vi "CH3_Save_Header_Python.vi"() -> ()   [LabVIEW 2018]
uses:
  RxTx/RxTx.lvclass
  Save Image/Save Image.lvclass
panel:
  out "error out":errorcluster
  in  "Save Image out":refnum<class "Save Image.lvclass">
  in  "RxTx.lvclass":refnum<class "RxTx.lvclass">
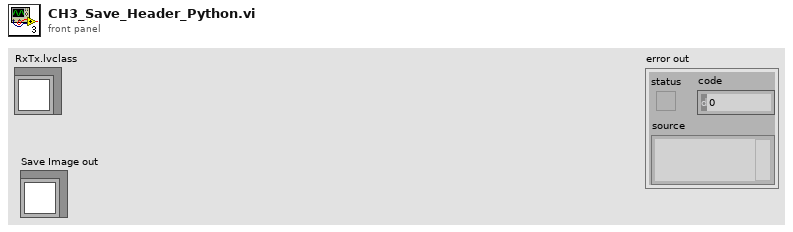
[diagram p1: front panel]
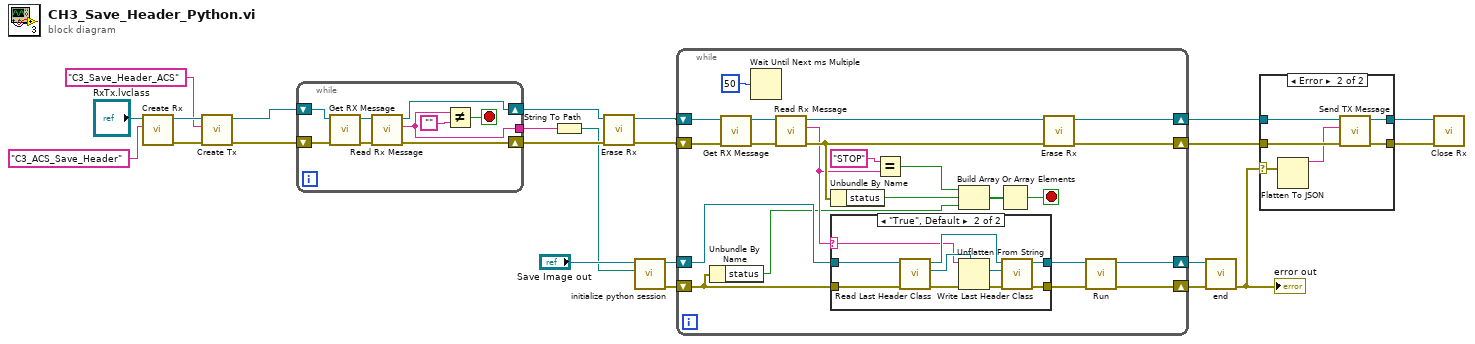
[diagram p0: block diagram]
diagram:
  n1 = call "Create Rx.vi"("Reader Name"="C3_ACS_Save_Header", "RxTx in"="RxTx.lvclass") -> ("error out"=w2:errorcluster, "RxTx out"=w5:refnum<class "RxTx.lvclass">)  [unwired: 8 in]
  n2 = call "Create Tx.vi"("error in (no error)"=w2, "Writer Name"="C3_Save_Header_ACS" ("Reader Name"), "RxTx in"=w5) -> ("error out"=w3:errorcluster, "RxTx out"=w4:refnum<class "RxTx.lvclass">)  [unwired: 7 in]
  n3 = while {
    shift-right: [w30] -> w16
    shift-left: w3 -> [w32]
    shift-right: [w29] -> w13
    shift-left: w4 -> [w27]
    tunnel: [w24] -> w11
    stop <- w25 stop-if-true
    n4 = call "Get RX Message.vi"("error in (no error)"=w32, "RxTx in"=w27) -> ("error out"=w31:errorcluster, "RxTx out"=w28:refnum<class "RxTx.lvclass">)  [unwired: 8 in]
    n5 = call "Read Rx Message.vi"("error in (no error)"=w31, "RxTx in"=w28) -> ("error out"=w30:errorcluster, "Rx Message"=w24:string, "RxTx out"=w29:refnum<class "RxTx.lvclass">)  [unwired: 7 in]
    n6 = Not Equal?(x=w24, y="") -> (x != y?=w25:bool)
  }
  n7 = String To Path(string=w11) -> (path=w12:path)
  n8 = call "Erase Rx.vi"("error in (no error)"=w16, "RxTx in"=w13) -> ("error out"=w15:errorcluster, "RxTx out"=w14:refnum<class "RxTx.lvclass">)  [unwired: 8 in]
  n9 = call "initialize python session.vi"("Optional Path to Python.exe"=w12, "Save Image in"="Save Image out") -> ("error out"=w20:errorcluster, "Save Image out"=w21:refnum<class "Save Image.lvclass">)  [unwired: 8 in]
  n10 = while {
    shift-right: [w42] -> w9
    shift-left: w15 -> [w53]
    shift-right: [w43] -> w10
    shift-left: w14 -> [w54]
    shift-right: [w45] -> w18
    shift-left: w21 -> [w47]
    shift-right: [w46] -> w17
    shift-left: w20 -> [w38]
    stop <- w33 stop-if-true
    n11 = Unbundle By Name(w38) -> ("status"=w37:bool)
    n12 = call "Get RX Message.vi"("error in (no error)"=w53, "RxTx in"=w54) -> ("error out"=w51:errorcluster, "RxTx out"=w52:refnum<class "RxTx.lvclass">)  [unwired: 8 in]
    n13 = Wait Until Next ms Multiple(millisecond multiple=u32 50) -> ()  [unwired: 1 out]
    n14 = call "Read Rx Message.vi"("error in (no error)"=w51, "RxTx in"=w52) -> ("error out"=w41:errorcluster, "Rx Message"=w39:string, "RxTx out"=w44:refnum<class "RxTx.lvclass">)  [unwired: 7 in]
    n15 = Unbundle By Name(w41) -> ("status"=w36:bool)
    n16 = case shown="\"True\", Default" w39 {
      selector: w39 -> [_ w57]
      tunnel: [w56 w58] -> w49
      tunnel: [w55 w59] -> w48
      tunnel: w38 -> [w55 w62]
      tunnel: w47 -> [w56 w63]
      frame "", "STOP" {
      }
      frame "True", Default {
        n17 = call "Read Last Header Class.vi"("error in (no error)"=w62, "Save Image in"=w63) -> ("error out"=w61:errorcluster, "Simulated_Header.lvclass"=w66:refnum<class "Simulated_Header.lvclass">, "Save Image out"=w64:refnum<class "Save Image.lvclass">)  [unwired: 7 in]
        n18 = Unflatten From String(type=w66, binary string=w57, error in (no error)=w61) -> (value=w65:refnum<class "Simulated_Header.lvclass">, error out=w60:errorcluster)  [unwired: 2 in, 1 out]
        n19 = call "Write Last Header Class.vi"("error in (no error)"=w60, "Simulated_Header.lvclass"=w65, "Save Image in"=w64) -> ("error out"=w59:errorcluster, "Save Image out"=w58:refnum<class "Save Image.lvclass">)  [unwired: 7 in]
      }
    }
    n20 = Equal?(x="STOP" ("Reader Name"), y=w39) -> (x = y?=w35:bool)
    n21 = Build Array(w35, w36, w37) -> (w34:bool[])
    n22 = Or Array Elements(Boolean array=w34) -> (logical OR=w33:bool)
    n23 = call "Erase Rx.vi"("error in (no error)"=w41, "RxTx in"=w44) -> ("error out"=w42:errorcluster, "RxTx out"=w43:refnum<class "RxTx.lvclass">)  [unwired: 8 in]
    n24 = call "Run.vi"("error in (no error)"=w48, "Save Image in"=w49) -> ("error out"=w46:errorcluster, "Save Image out"=w45:refnum<class "Save Image.lvclass">)  [unwired: 8 in]
  }
  n25 = call "end.vi"("error in (no error)"=w17, "Save Image in"=w18) -> ("error out"=w6:errorcluster)  [unwired: 8 in, 1 out]
  "error out" <- w6
  n26 = case shown="Error" w6 {
    selector: w6 -> [_ w70]
    tunnel: w10 -> [w68 w74]
    tunnel: w9 -> [w67 w73]
    tunnel: [w67 w72] -> w8
    tunnel: [w68 w71] -> w7
    frame No Error {
    }
    frame Error {
      n27 = Flatten To JSON(anything=w70) -> (JSON string=w69:string)  [unwired: 2 in, 1 out]
      n28 = call "Send TX Message.vi"("error in (no error)"=w73, "element"=w69, "RxTx in"=w74) -> ("error out"=w72:errorcluster, "RxTx out"=w71:refnum<class "RxTx.lvclass">)  [unwired: 7 in]
    }
  }
  n29 = call "Close Rx.vi"("error in (no error)"=w8, "RxTx in"=w7) -> ()  [unwired: 8 in, 2 out]
